vi "Send Write Setup.vi"(8 "error in (no error)":errorcluster, 11 "Channel in":refnum<class "Channel.lvclass">) -> (0 "error out":errorcluster, 3 "Channel out":refnum<class "Channel.lvclass">)   [LabVIEW 2018, in "Channel.lvclass"]
uses:
  Channel.lvclass
  Channel.lvclass/Channel.ctl
  Interface/Interface.lvclass
  RxTx/RxTx.lvclass
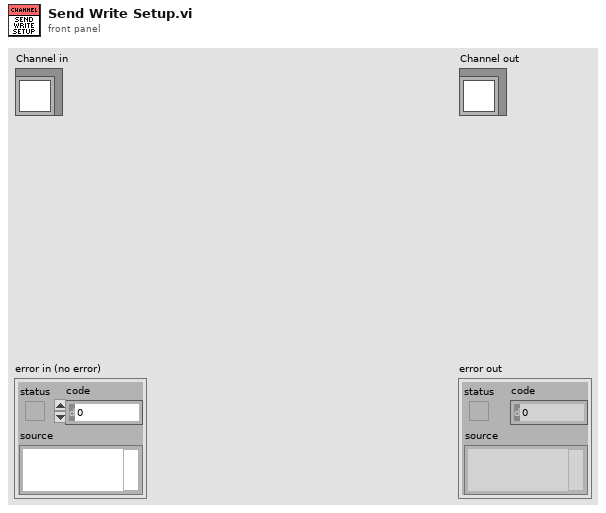
[diagram p1: front panel]
types:
  T1 = typedef "Shutter_mode typedef.ctl" = enum16{"Auto", "Open", "Close", "N/A (3)", "Open FVB Series", "Open Any Series"}
  T2 = typedef "ReadMode_mode typedef.ctl" = enum16{"Full Vertical Binning", "Multi-Track", "Random-Track", "Single-Track", "Image"}
  T3 = typedef "AcquisitionMode_mode typedef.ctl" = enum16{"Reserved (0)", "Single Scan", "Accumulate", "Kinetics", "Fast Kinetics", "Run Till Abort", "Reserved (6)", "Reserved (7)", "Reserved (8)", "Time Delayed Integration"}
  T4 = cluster{"PREAMP":enum16{"Gain 1", "Gain 2"}, "READOUT_RATE":enum16{"30 MHz", "20 MHz", "10 MHz", "1 MHz"}, "EM_GAIN":u16, "VBIN":u16, "INITIAL_LINE":u16, "INITIAL_COLUMN":u16, "FINAL_LINE":u16, "FINAL_COLUMN":u16, "TRIGGER_MODE":enum16{"Internal", "External", "N/A", "N/A_1", "N/A_2", "N/A_3", "External Start"}, "HBIN":u16, "SHUTTER_TTL":enum16{"TTL Low", "TTL High"}, "SHUTTER_MODE":T1, "SHUTTER_OPENING_TIME":u16, "SHUTTER_CLOSING_TIME":u16, "VERTICAL_SHIFT_SPEED":u16, "READ_MODE":T2, "FRAME_TRANSFER":bool, "VERTICAL_CLOCK_VOLTAGE":enum16{"0", "+1", "+2", "+3", "+4"}, "ACQUISITION_MODE":T3, "AD_CHANNEL":u16, "EM_MODE":enum16{"Electron Multiplying", "Conventional"}}
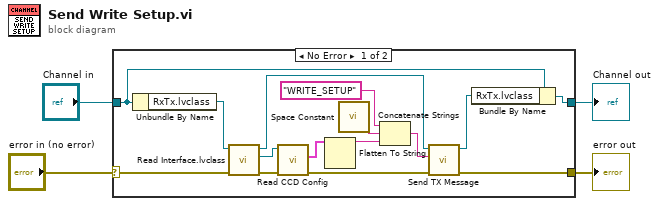
[diagram p0: block diagram]
diagram:
  n1 = case shown="No Error" "error in (no error)" {
    selector: "error in (no error)" -> [w19 w21]
    tunnel: [w8 w21] -> w3
    tunnel: [w9 w20] -> w1
    tunnel: "Channel in" -> [w10 w20]
    frame No Error {
      n2 = Unbundle By Name(w10) -> ("RxTx.lvclass"=w18:refnum<class "RxTx.lvclass">)
      n3 = call "Read Interface.lvclass.vi"("error in (no error)"=w19, "RxTx in"=w18) -> ("error out"=w16:errorcluster, "Interface.lvclass"=w17:refnum<class "Interface.lvclass">, "RxTx out"=w6:refnum<class "RxTx.lvclass">)  [unwired: 7 in]
      n4 = call "Read CCD Config.vi"("error in (no error)"=w16, "Interface in"=w17) -> ("error out"=w5:errorcluster, "CCD Config"=w15:T4)  [unwired: 7 in, 1 out]
      n5 = Flatten To String(anything=w15) -> (data string=w13:string)  [unwired: 3 in, 2 out]
      n6 = call <vilib>:"Space Constant.vi"() -> ("String"=w12:string)
      n7 = Concatenate Strings("WRITE_SETUP" ("string"), w12, w13) -> (w7:string)
      n8 = call "Send TX Message.vi"("error in (no error)"=w5, "element"=w7, "RxTx in"=w6) -> ("error out"=w8:errorcluster, "RxTx out"=w11:refnum<class "RxTx.lvclass">)  [unwired: 7 in]
      n9 = Bundle By Name(cluster=w10, "RxTx.lvclass"=w11) -> (w9:refnum<class "Channel.lvclass">)
    }
    frame Error {
    }
  }
  "error out" <- w3
  "Channel out" <- w1
